vi "GetLogStr.vi"(8 "error in (no error)":errorcluster, 10 "LogRecord in":refnum<class "LogRecord.lvclass">, 11 "FileHandler in":refnum<class "RotateFileHandler.lvclass">) -> (0 "error out":errorcluster, 2 "LogLine":string, 3 "FileHandler out":refnum<class "RotateFileHandler.lvclass">)   [LabVIEW 2024, in "RotateFileHandler.lvclass"]
uses:
  RotateFileHandler.lvclass
  <vilib>/Hampel Software Engineering/HSE Logger/LogRecord/LogRecord.lvclass
  RotateFileHandler.lvclass/RotateFileHandler.ctl
  <vilib>/Hampel Software Engineering/HSE Logger/Formatter/Formatter.lvclass
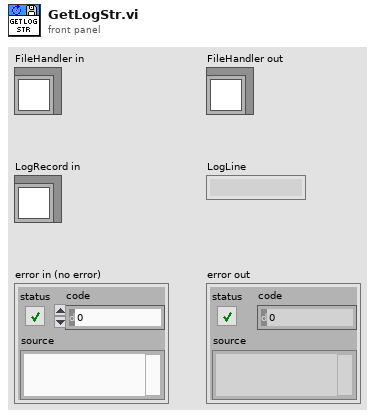
[diagram p1: front panel]
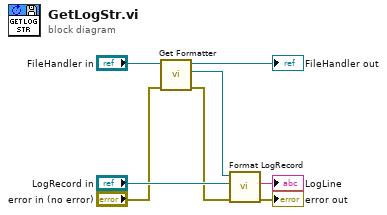
[diagram p0: block diagram]
diagram:
  n1 = call "Get Formatter.vi"("error in"="error in (no error)", "FileHandler"="FileHandler in") -> ("error out"=w3:errorcluster, "Formatter"=w7:refnum<class "Formatter.lvclass">, "FileHandler out"=→"FileHandler out":refnum<class "RotateFileHandler.lvclass">)  [unwired: 7 in]
  n2 = call-dynamic "Format LogRecord.vi"("error in"=w3, "LogRecord"="LogRecord in", "Formatter in"=w7) -> ("error out"=→"error out":errorcluster, "LogLine"=→"LogLine":string)  [unwired: 7 in]
